vi "Encoded String To UTF-8.vi"(8 "error in (no error)":errorcluster, 10 "Encoded string":string, 11 "Encoding in":refnum<class "CConfig UTF-8-BOM Encoding.lvclass">) -> (0 "error out":errorcluster, 2 "UTF-8 string":string, 3 "Encoding out":refnum<class "CConfig UTF-8-BOM Encoding.lvclass">)   [LabVIEW 2013, in "CConfig UTF-8-BOM Encoding.lvclass"]
doc: "Copyright 2018, Carya Automatisering, Wiebe Walstra."
uses:
  CConfig UTF-8-BOM Encoding.lvclass
  <vilib>/Utility/error.llb/Error Cluster From Error Code.vi
  <vilib>/ErrorRing/Error Ring.xnode
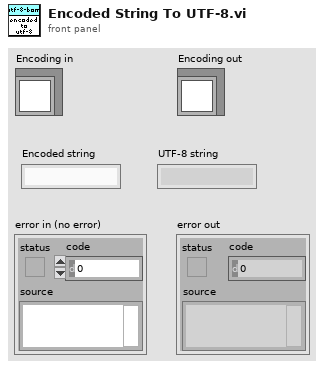
[diagram p1: front panel]
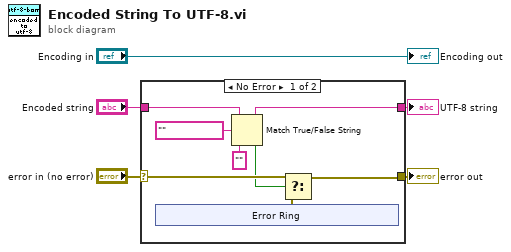
[diagram p0: block diagram]
diagram:
  n1 = case shown="No Error" "error in (no error)" {
    selector: "error in (no error)" -> [w9 w19]
    tunnel: [w8 w19] -> w3
    tunnel: "Encoded string" -> [w11 w20]
    tunnel: [w10 w20] -> w1
    frame No Error {
      n2 = xnode "Error Ring"() -> ("error out"=w6:errorcluster)
      n3 = Match True/False String(2:"" ("false string"), 3:"﻿" ("true string"), 4:w11) -> (0:w7:bool, 1:w10:string)
      n4 = Select(t=w9, s=w7, f=w6) -> (s? t:f=w8:errorcluster)
    }
    frame Error {
    }
  }
  "error out" <- w3
  "UTF-8 string" <- w1
  "Encoding out" <- "Encoding in"
